vi "Add Server.vi"(8 "error in (no error)":errorcluster, 11 "WebSocket Server Manager in":refnum<class "WebSocket Server Manager.lvclass">) -> (0 "error out":errorcluster, 3 "WebSocket Server Manager out":refnum<class "WebSocket Server Manager.lvclass">)   [LabVIEW 2016, in "WebSocket Actors.lvlib" / "WebSocket Server Manager.lvclass"]
uses:
  WebSocket Server Manager.lvclass
  WebSocket Server/WebSocket Server.lvclass
  <vilib>/ActorFramework/Actor/Actor.lvclass
  C:/Program Files (x86)/National Instruments/LabVIEW 2016/vi.lib/MGI/Monitored Actor/Monitored Actor/Monitored Actor/Monitored Actor.lvclass
  C:/Program Files (x86)/National Instruments/LabVIEW 2016/vi.lib/ActorFramework/Actor/Actor.lvclass
  WebSocket Server/typedefs/Listener Settings.ctl
  <vilib>/ActorFramework/Message Enqueuer/Message Enqueuer.lvclass
panel:
  in  "Subscriber Enqueuer":refnum<class "Message Enqueuer.lvclass">
  in  "Handshake timeout (5000 ms)":i32=5000
  in  "Listener Settings":T1={"resolve remote address (T)"=TRUE, "timeout ms (-1)"=-1, "net address"=0, "port"=6163}
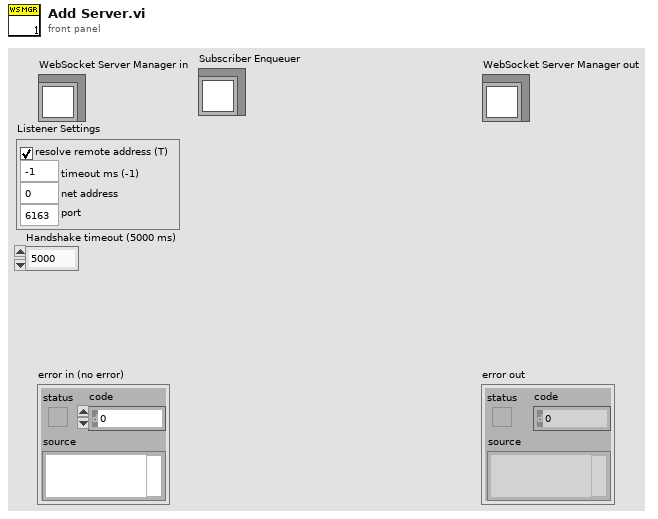
[diagram p1: front panel]
types:
  T1 = typedef "WebSocket Actors.lvlib/WebSocket Server.lvclass/Listener Settings.ctl" = cluster{"resolve remote address (T)":bool, "timeout ms (-1)":i32, "net address":u32, "port":u16}
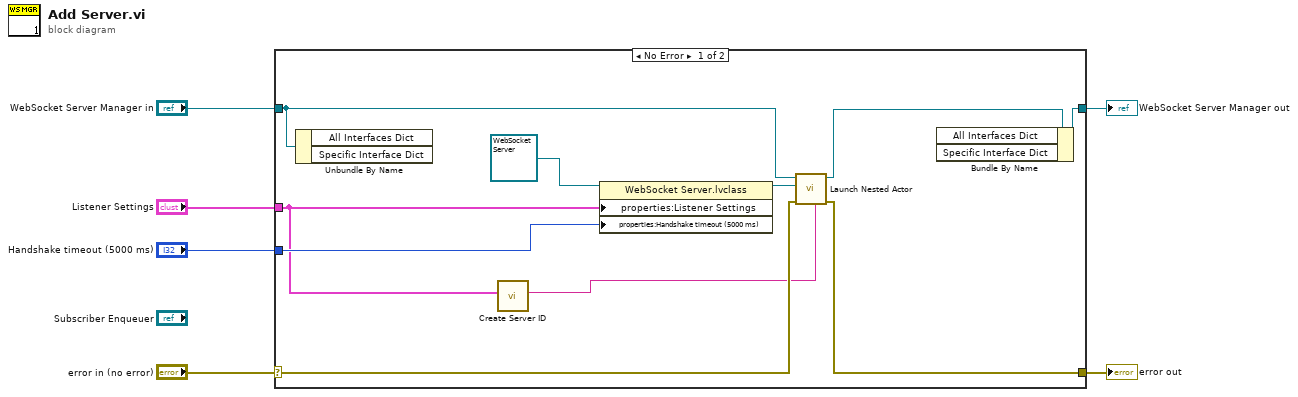
[diagram p0: block diagram]
diagram:
  n1 = case shown="No Error" "error in (no error)" {
    selector: "error in (no error)" -> [w13 w18]
    tunnel: [w12 w18] -> w5
    tunnel: [w11 w17] -> w3
    tunnel: "WebSocket Server Manager in" -> [w10 w17]
    tunnel: "Handshake timeout (5000 ms)" -> [w14 _]
    tunnel: "Listener Settings" -> [w8 _]
    frame No Error {
      n2 = Unbundle By Name(w10) -> ()  [unwired: 2 out]
      n3 = call "Create Server ID.vi"("Listener Settings"=w8) -> ("Server ID"=w7:string)  [unwired: 9 in]
      n4 = property class="WebSocket Server.lvclass"(reference=refnum<class "WebSocket Server.lvclass"> refnum ("WebSocket Actors.lvlib:WebSocket Server.lvclass"), "properties:Listener Settings"=w8, "properties:Handshake timeout (5000 ms)"=w14) -> (reference out=w15:refnum<class "WebSocket Server.lvclass">)  [unwired: 1 in, 1 out]
      n5 = call <vilib>:"Launch Nested Actor.vi"("Debug Alias"=w7, "error in (no error)"=w13, "Nested Actor"=w15, "Caller Actor in"=w10) -> ("error out"=w12:errorcluster, "Caller Actor out"=w9:refnum<class "WebSocket Server Manager.lvclass">)  [unwired: 5 in, 1 out]
      n6 = Bundle By Name(cluster=w9) -> (w11:refnum<class "WebSocket Server Manager.lvclass">)  [unwired: 2 in]
    }
    frame Error {
    }
  }
  "error out" <- w5
  "WebSocket Server Manager out" <- w3
